vi "ConfigAquisitionParam.vi"(4 "Requested Samples Per Pixel":u16, 5 "Downsample [0,1,2]":u8, 6 "ProcessCompletionDelay (us)":sgl, 7 "vi/nGenTrig":bool, 8 "error in":errorcluster, 9 "AvgCount_powerOf2":i16, 10 "Delay (us)":sgl, 11 "FPGA VI Reference In":T1) -> (0 "error out":errorcluster, 2 "Read Size (Host)":u16, 3 "FPGA VI Reference Out":T1)   [LabVIEW 2020]
uses:
  Controls/FPGA VI Reference.ctl
  <vilib>/Utility/error.llb/Error Cluster From Error Code.vi
  <vilib>/rvi/errors/niLvFpgaAdjustHostInterfaceError.vi
  <vilib>/rvi/interface/nirviReadWriteControl/nirviReadWriteControl.xnode
  NiFpgaLv.dll
  <vilib>/rvi/interface/Simulation/niFpgaSimulationCallBeginRW.vi
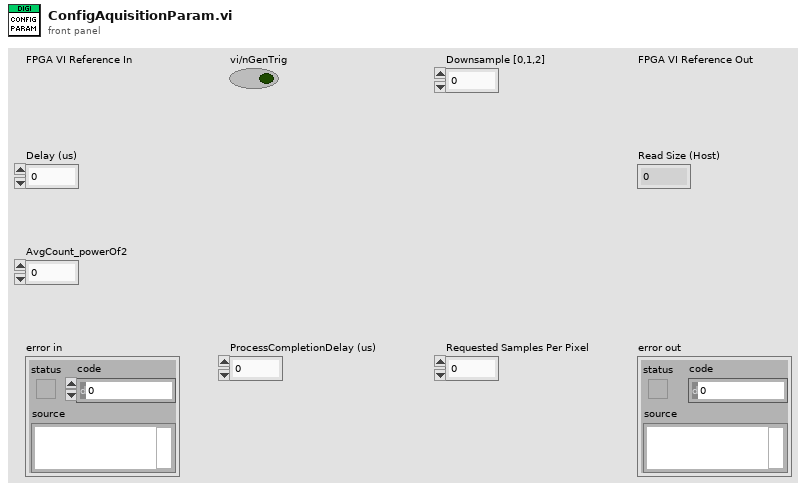
[diagram p1: front panel]
types:
  T1 = typedef "FPGA VI Reference.ctl" = refnum<k20>
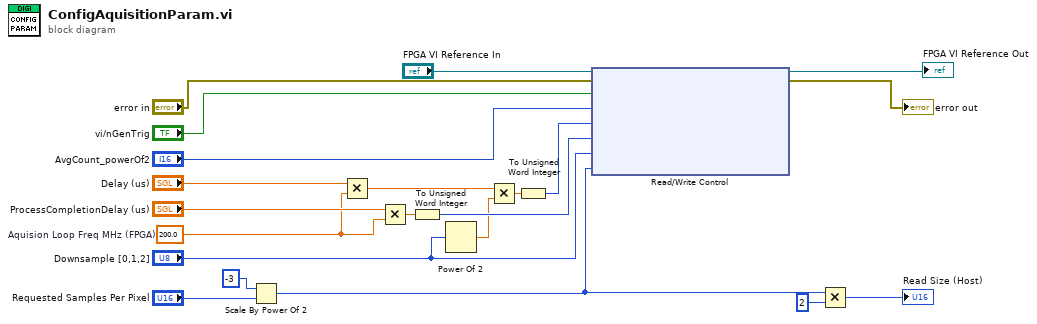
[diagram p0: block diagram]
diagram:
  w15 = sgl 200.0  # Aquision Loop Freq MHz (FPGA)
  n1 = Scale By Power Of 2(n=i16 -3, x="Requested Samples Per Pixel") -> (x*2^n=w9:u16)
  n2 = Multiply(x="Delay (us)", y=w15) -> (x*y=w13:sgl)
  n3 = Multiply(x="ProcessCompletionDelay (us)", y=w15) -> (x*y=w14:sgl)
  n4 = To Unsigned Word Integer(number=w14) -> (unsigned 16bit integer=w12:u16)
  n5 = Power Of 2(x="Downsample [0,1,2]") -> (2^x=w4:dbl)
  n6 = Multiply(x=w13, y=w4) -> (x*y=w5:dbl)
  n7 = To Unsigned Word Integer(number=w5) -> (unsigned 16bit integer=w3:u16)
  n8 = xnode "Read/Write Control"("FPGA VI Reference In"="FPGA VI Reference In", "error in"="error in", "vi/nGenTrig"="vi/nGenTrig", "AvgCount_powerOf2"="AvgCount_powerOf2", "Delay Cycles"=w3, "WaitForWave Completion [cycles]"=w12, "DS"="Downsample [0,1,2]", "Samples Per Trigger"=w9) -> ("FPGA VI Reference Out"=→"FPGA VI Reference Out":T1, "error out"=→"error out":errorcluster)
  n9 = Multiply(x=w9, y=u16 2) -> (x*y=→"Read Size (Host)":u16)
